vi "Edit Icon.vi"(8 "error in (no error)":errorcluster, 10 "VI Refnum in":refnum<vi>, 11 "Model in":refnum<class "Model.lvclass">) -> (0 "error out":errorcluster, 3 "Model out":refnum<class "Model.lvclass">)   [LabVIEW 2015, in "Model.lvlib" / "Model.lvclass"]
uses:
  Model.lvclass
  <vilib>/LabVIEW Icon API/LabVIEW Icon API.lvlib
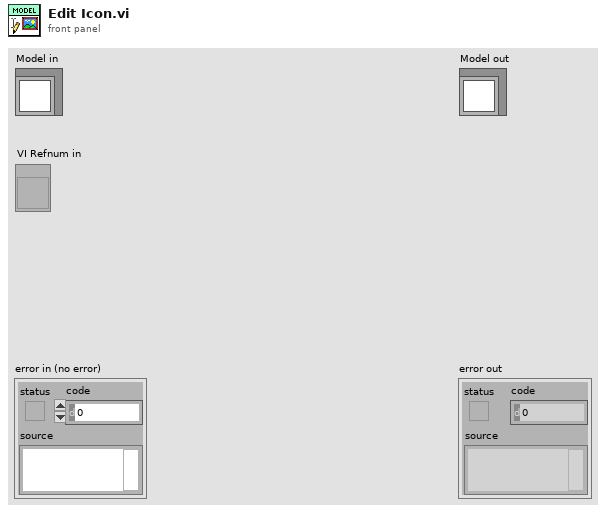
[diagram p1: front panel]
types:
  T1 = typedef "Model.lvlib/VI Infomation.ctl" = cluster{"Name":string, "Description":string, "Icon":picture}
  T2 = typedef "imagedata.ctl" = cluster{"image type":i32, "image depth":i32, "image":u8[], "mask":u8[], "colors":u32[], "Rectangle":cluster{"left":i16, "top":i16, "right":i16, "bottom":i16}}
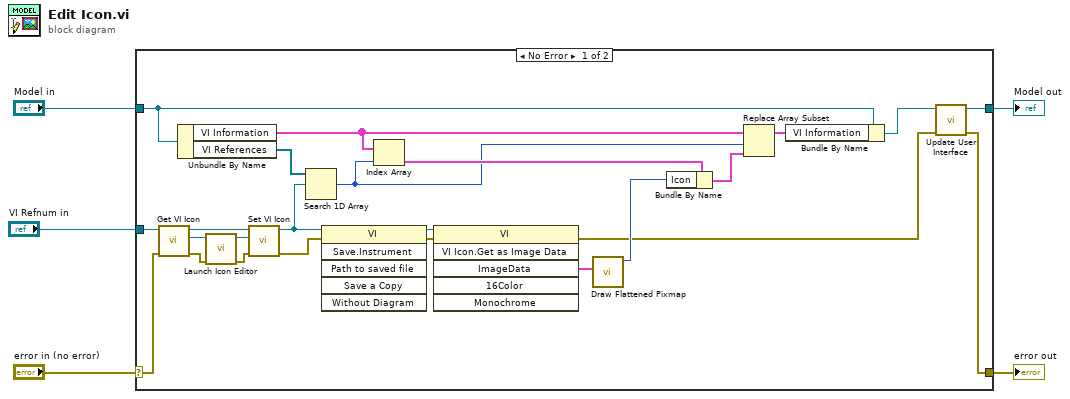
[diagram p0: block diagram]
diagram:
  n1 = case shown="No Error" "error in (no error)" {
    selector: "error in (no error)" -> [w24 w31]
    tunnel: [w22 w31] -> w4
    tunnel: [w23 w30] -> w2
    tunnel: "Model in" -> [w15 w30]
    tunnel: "VI Refnum in" -> [w20 _]
    frame No Error {
      n2 = call <vilib>:"Get VI Icon.vi"("error in (no error)"=w24, "VI Refnum in"=w20) -> ("error out"=w25:errorcluster, "Icon"=w28:refnum<class "Icon.lvclass">, "VI Refnum out"=w29:refnum<vi>)  [unwired: 7 in]
      n3 = Unbundle By Name(w15) -> ("VI Information"=w13:T1[], "VI References"=w8:refnum<vi>[])
      n4 = call <vilib>:"Launch Icon Editor.vi"("error in (no error)"=w25, "Icon in"=w28) -> ("error out"=w26:errorcluster, "Icon out"=w27:refnum<class "Icon.lvclass">)  [unwired: 7 in, 1 out]
      n5 = call <vilib>:"Set VI Icon.vi"("error in (no error)"=w26, "Icon"=w27, "VI Refnum in"=w29) -> ("error out"=w21:errorcluster, "VI Refnum out"=w19:refnum<vi>)  [unwired: 7 in]
      n6 = Search 1D Array(1D array=w8, element=w19) -> (index of element=w7:i32)  [unwired: 1 in]
      n7 = invoke class="VI" method="Save.Instrument"(reference=w19, error in=w21) -> (reference out=w16:refnum<vi>, error out=w17:errorcluster)  [unwired: 4 in, 4 out]
      n8 = Index Array(array=w13, index=w7) -> (element=w12:T1)
      n9 = invoke class="VI" method="VI Icon.Get as Image Data"(reference=w16, error in=w17) -> (error out=w6:errorcluster, "ImageData"=w18:T2)  [unwired: 4 in, 4 out]
      n10 = call <vilib>:"Draw Flattened Pixmap.vi"("image data"=w18) -> ("new picture"=w11:picture)  [unwired: 8 in]
      n11 = Bundle By Name(cluster=w12, "Icon"=w11) -> (w10:T1)
      n12 = Replace Array Subset(array=w13, new element=w10, index=w7) -> (w9:T1[])
      n13 = Bundle By Name(cluster=w15, "VI Information"=w9) -> (w14:refnum<class "Model.lvclass">)
      n14 = call "Update User Interface.vi"("error in (no error)"=w6, "Model in"=w14) -> ("error out"=w22:errorcluster, "Model out"=w23:refnum<class "Model.lvclass">)  [unwired: 8 in]
    }
    frame Error {
    }
  }
  "error out" <- w4
  "Model out" <- w2
